vi "EllipRegionConstraint_New.vi"(6 "Constraint Data Cluster":variant, 8 "Rotation":T1={"VALUE"=0.0, "COS"=1.0, "SIN"=0.0} {"SIN" format="%13.4f"; "COS" format="%13.4f"; "VALUE" format="%13.4f"}, 9 "Y Width":dbl, 10 "X Width":dbl, 11 "Center":T2 {"Y" format="%14.3f"; "X" format="%14.3f"}) -> (3 "ELLIP_REGION_CONSTRAINT":T3={"Center"={"X"=0.0, "Y"=0.0}, "Radii"={"X"=0.0, "Y"=0.0}, "Constraint"=variant, "Constraint Type"=enum."DIFF DRIVE KINEMATICS"} {"Radii"."Y" format="%14.3f"; "Radii"."X" format="%14.3f"; "Center"."Y" format="%14.3f"; "Center"."X" format="%14.3f"})   [LabVIEW 2019, in "Trajectory_Library.lvlib"]
doc: "Constructs a differential drive dynamics constraint.\n\n\nParameters:\n - MaxSpeed - Max speed (meters/sec)\n - DiffDriveKinematics - Diff Drive Kinematics data structure\n\nReturns\n - DiffDriveKineConstraint - Constraint data structure."
uses:
  Trajectory_Library.lvlib
  TypeDef/TRAJ_CONSTRAINT_ELLIP_REGION.ctl
  TRANSLATION2D.ctl
  TypeDef/TRAJ_CONSTRAINT_TYPES_ENUM.ctl
  <vilib>/Utility/Data Type/Get Type Information.vi
  ROTATION2D.ctl
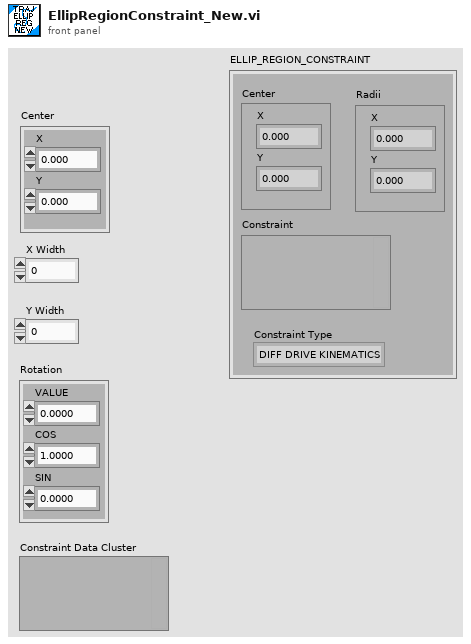
[diagram p1: front panel]
types:
  T1 = typedef "Trajectory_Library.lvlib/ROTATION2D.ctl" = cluster{"VALUE":dbl, "COS":dbl, "SIN":dbl}
  T2 = typedef "Trajectory_Library.lvlib/TRANSLATION2D.ctl" = cluster{"X":dbl, "Y":dbl}
  T3 = typedef "Trajectory_Library.lvlib/TRAJ_CONSTRAINT_ELLIP_REGION.ctl" = cluster{"Center":T2, "Radii":T2, "Constraint":variant, "Constraint Type":T4}
  T4 = typedef "Trajectory_Library.lvlib/TRAJ_CONSTRAINT_TYPES_ENUM.ctl" = enum16{"UNDEFINED", "DIFF DRIVE KINEMATICS", "DIFF DRIVE VOLTAGE", "CENTRIPITAL ACCEL", "MECA DRIVE KINEMATICS", "SWERVE DRIVE KINEMATICS"}
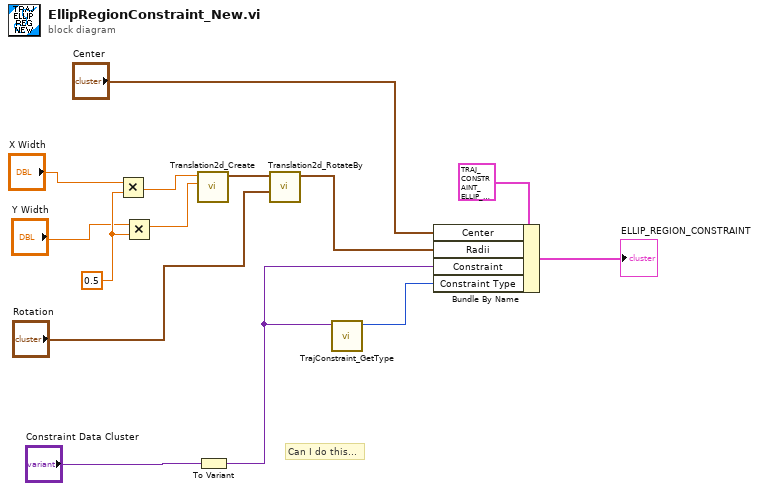
[diagram p0: block diagram]
diagram:
  w8 = 0.5 ("y")
  # "Can I do this..."
  n1 = Multiply(x="X Width", y=w8) -> (x*y=w5:dbl)
  n2 = Multiply(x="Y Width", y=w8) -> (x*y=w4:dbl)
  n3 = call "Translation2d_Create.vi"("Y"=w4, "X"=w5) -> ("TRANSLATION"=w3:T2)  [unwired: 9 in]
  n4 = To Variant(anything="Constraint Data Cluster") -> (Variant=w10:variant)
  n5 = call "Translation2d_RotateBy.vi"("other Rotation"="Rotation", "In Translation"=w3) -> ("Out Translation"=w1:T2)  [unwired: 9 in]
  n6 = call "TrajConstraint_GetType.vi"("Trajectory Constraint"=w10) -> ("Trajectory Constraint Type"=w9:T4)  [unwired: 9 in, 1 out]
  n7 = Bundle By Name(cluster=T3 {"Center"={"X"=0.0, "Y"=0.0}, "Radii"={"X"=0.0, "Y"=0.0}, "Constraint"=variant, "Constraint Type"=enum."DIFF DRIVE KINEMATICS"} ("ELLIP_REGION_CONSTRAINT"), "Center"="Center", "Radii"=w1, "Constraint"=w10, "Constraint Type"=w9) -> (→"ELLIP_REGION_CONSTRAINT":T3)
